vi "regress_RTD.vi"(0 "R (Ohm)":dbl=100.0, 5 "R0 (Ohm)":dbl=100.0, 7 "A (K^-1)":dbl, 9 "B (K^-2)":dbl, 11 "C (K^-3)":dbl, 12 "dev":dbl) -> (8 "T (K)":dbl)   [LabVIEW 2018]
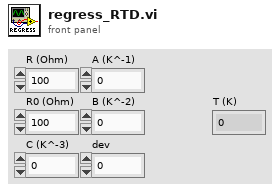
[diagram p1: front panel]
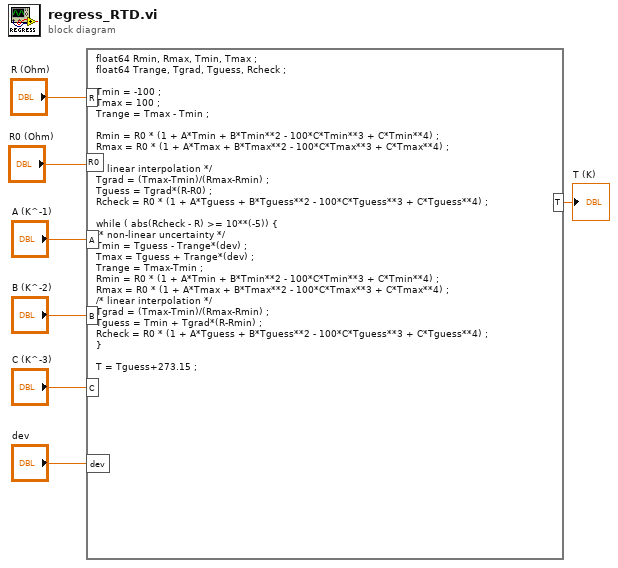
[diagram p0: block diagram]
diagram:
  n1 = formula code="float64 Rmin, Rmax, Tmin, Tmax ;\nfloat64 Trange, Tgrad, Tguess, Rcheck ;\n\nTmin = -100 ;\nTmax = 100 ;\nTrange = Tmax - Tmin ;\n\nRmin = R0 * (1 + A*Tmin + B*Tmin**2 - 100*C*Tmin**3 + C*Tmin**4) ;\nRmax = R0 * (1 + A*Tmax + B*Tmax**2 - 100*C*Tmax**3 + C*Tmax**4) ;\n\n/* linear interpolation */\nTgrad = (Tmax-Tmin)/(Rmax-Rmin) ;\nTguess = Tgrad*(R-R0) ;\nRcheck = R0 * (1 + A*Tguess + B*Tguess**2 - 100*C*Tguess**3 + C*Tguess**4) ;\n\nwhile ( abs(Rcheck - R) >= 10**(-5)) {\n/* non-linear uncertainty */\nTmin = Tguess - Trange*(dev) ;\nTmax = Tguess + Trange*(dev) ;\nTrange = Tmax-Tmin ;\nRmin = R0 * (1 + A*Tmin + B*Tmin**2 - 100*C*Tmin**3 + C*Tmin**4) ;\nRmax = R0 * (1 + A*Tmax + B*Tmax**2 - 100*C*Tmax**3 + C*Tmax**4) ;\n/* linear interpolation */\nTgrad = (Tmax-Tmin)/(Rmax-Rmin) ;\nTguess = Tmin + Tgrad*(R-Rmin) ;\nRcheck = R0 * (1 + A*Tguess + B*Tguess**2 - 100*C*Tguess**3 + C*Tguess**4) ;\n}\n\nT = Tguess+273.15 ;"("R0"="R0 (Ohm)", "A"="A (K^-1)", "B"="B (K^-2)", "C"="C (K^-3)", "R"="R (Ohm)", "dev"="dev") -> ("T"=→"T (K)":dbl)
